vi "adam-DO-channel-command-builder.vi"(8 "Stop All":bool, 9 "Channel Active":bool, 10 "Channel Number":dbl=1.0, 11 "Device Address":dbl=1.0) -> (0 "Desired State":bool, 3 "concatenated command":string)   [LabVIEW 2021]
panel:
  out "Data String":string
  out "Device Address":string
  out "Channel Number":string
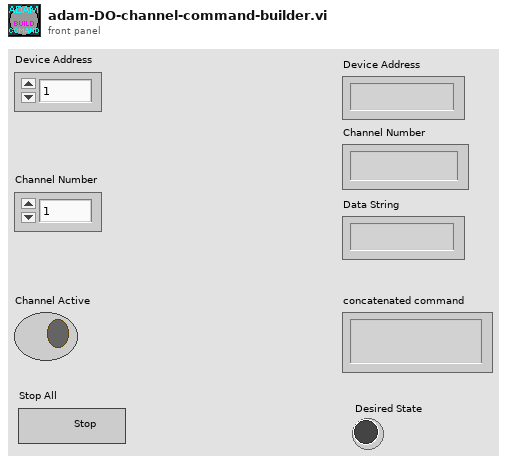
[diagram p1: front panel]
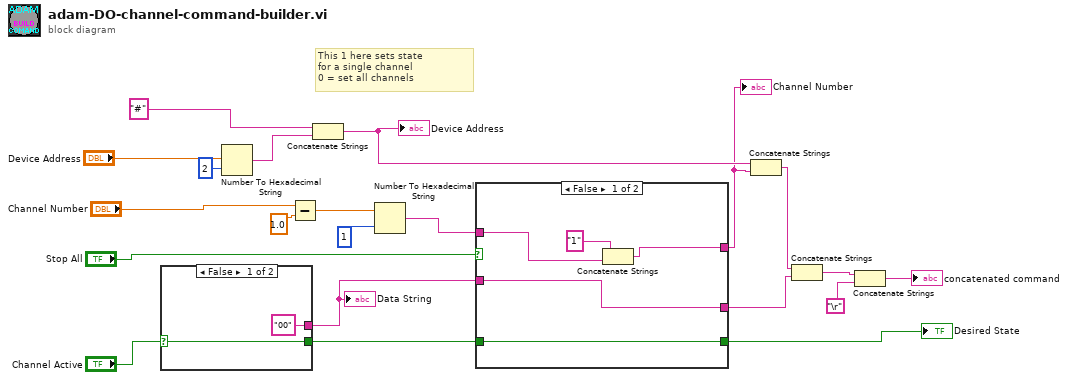
[diagram p0: block diagram]
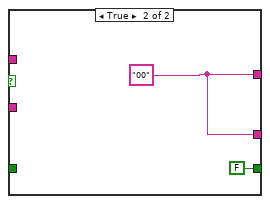
[diagram p2: hidden frame]
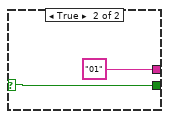
[diagram p3: hidden frame]
diagram:
  # "This 1 here sets state\nfor a single channel\n0 = set all channels"
  n1 = case shown="False" "Channel Active" {
    selector: "Channel Active" -> [w22 w24]
    tunnel: ["00" "01"] -> w6
    tunnel: [w22 w24] -> w1
    frame False {
    }
    frame True {
    }
  }
  "Data String" <- w6
  n2 = Number To Hexadecimal String(1:i16 2 ("width (-)"), 2:"Device Address") -> (0:w8:string)
  n3 = Subtract(x="Channel Number", y=1.0) -> (x-y=w18:dbl)
  n4 = Concatenate Strings("#" ("string"), w8) -> (w11:string)
  "Device Address" <- w11
  n5 = Number To Hexadecimal String(1:i16 1 ("width (-)"), 2:w18) -> (0:w21:string)
  n6 = case shown="False" "Stop All" {
    tunnel: w21 -> [w29 _]
    tunnel: [w28 w32] -> w4
    tunnel: w6 -> [w27 _]
    tunnel: [w27 w32] -> w3
    tunnel: [w26 FALSE] -> w2
    tunnel: w1 -> [w26 _]
    frame False {
      n7 = Concatenate Strings("1" ("string"), w29) -> (w28:string)
    }
    frame True {
      w32 = "00"
    }
  }
  "Desired State" <- w2
  "Channel Number" <- w4
  n8 = Concatenate Strings(w11, w4) -> (w16:string)
  n9 = Concatenate Strings(w16, w3) -> (w17:string)
  n10 = Concatenate Strings(w17, "\r") -> (→"concatenated command":string)
